vi "Two Lambda ZUP control panel.vi"() -> ()   [LabVIEW 2010]
uses:
  <vilib>/Instr/_visa.llb/VISA Configure Serial Port (Instr).vi
panel:
  in  "stop":bool
  out "Connected 2":bool
  out "Connected 1":bool
  in  "Run 2":bool
  in  "Run 1":bool
  out "read Lambda 2":string
  out "Code 2":string
  in  "Command 2":T1(ring)
  in  "Auxiliary Paramerter 2":dbl min=0.0 max=20.0 step=0.1
  out "read Lambda 1":string
  out "Code 1":string
  in  "Command 1":T1(ring)
  in  "Auxiliary Paramerter 1":dbl min=0.0 max=20.0 step=0.1
  in  "VISA resource name":refnum<visa-resource-name>
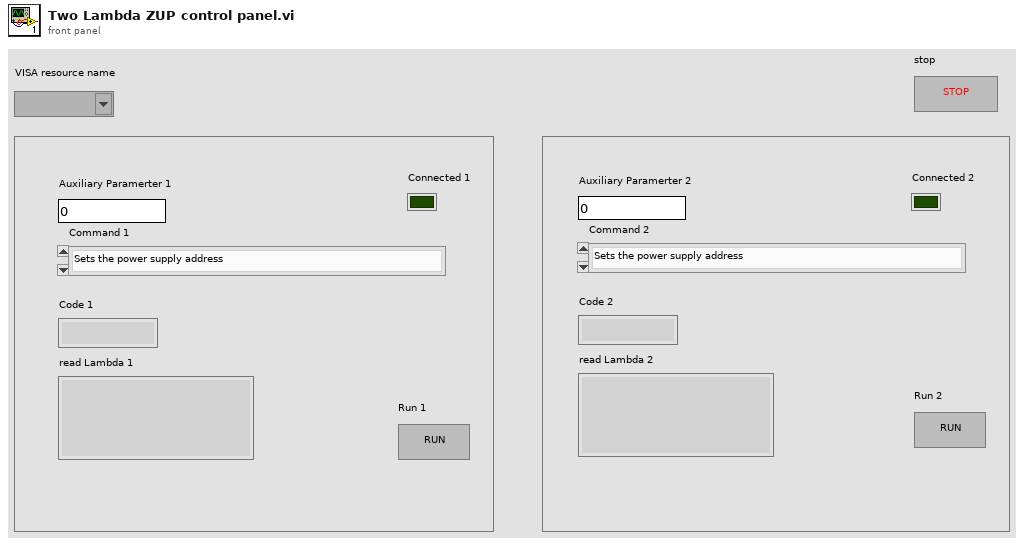
[diagram p1: front panel]
types:
  T1 = enum16{"Sets the power supply address", "Clears the communication buffer and the following registers", "Sets the power supply to local or remote mode", "Returns the remote/local setting", "Returns the power supply model identification", "Returns the software version", "Sets the output voltage value", "Returns the string SV (Set Voltage)", "Returns the string AV (Actual Voltage)", "Sets the output current in Ampers", "Returns the string SA (Set Amper)", "Returns the string AA (Actual Amper)", "Sets the output to On or Off", "Returns followed by the output On/Off status", "Sets the Foldback protection to On or Off", "Returns FD followed by the Foldback protection status", "Sets the over-voltage protection level in volts", "Returns the string OP  over-voltage protection value", "Sets the under-voltage protection limits in volts", "Returns the string UP under-voltage protection value", "Sets the auto-restart mode to On or Off", "Returns the string AS auto-restart mode status"}
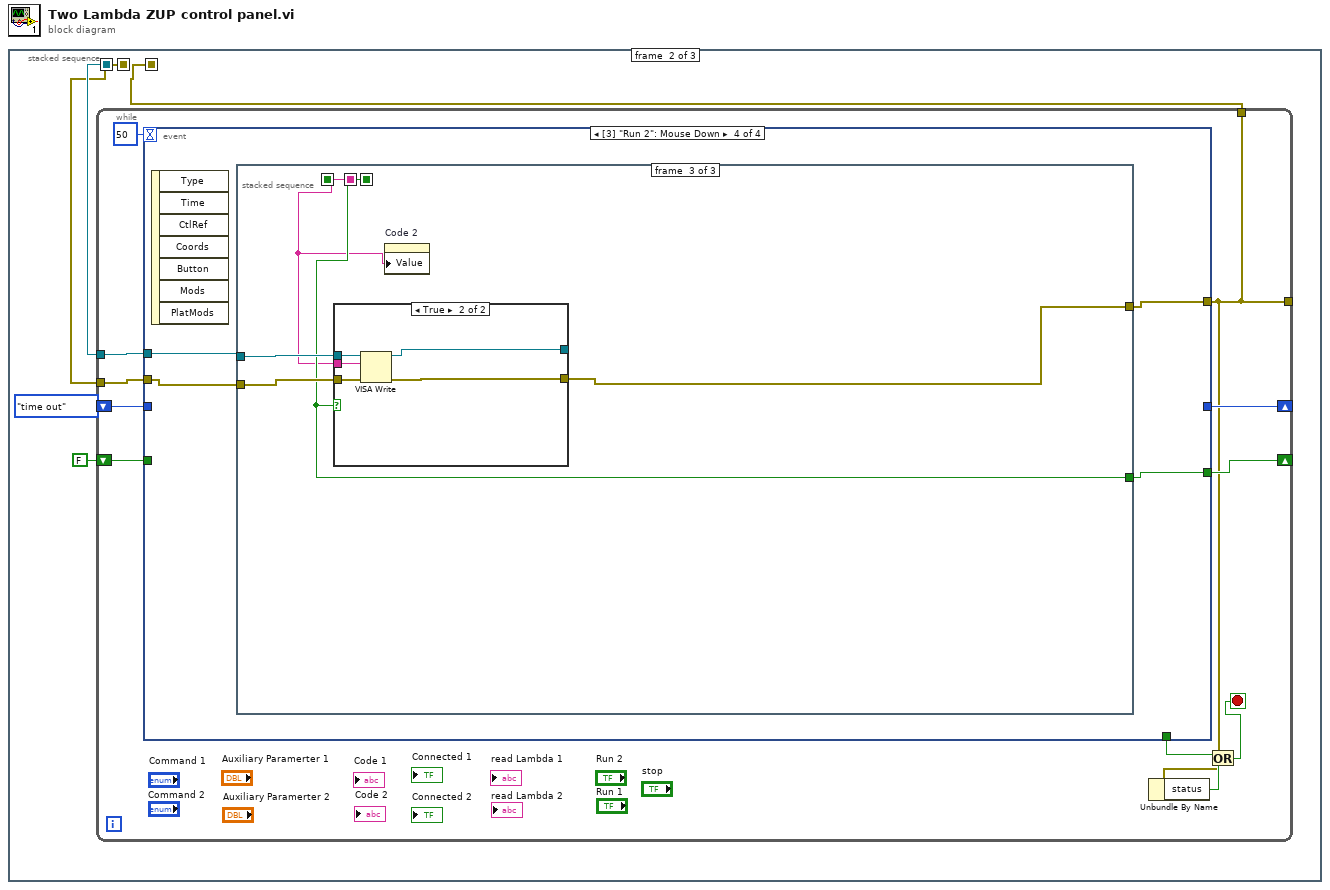
[diagram p0: block diagram]
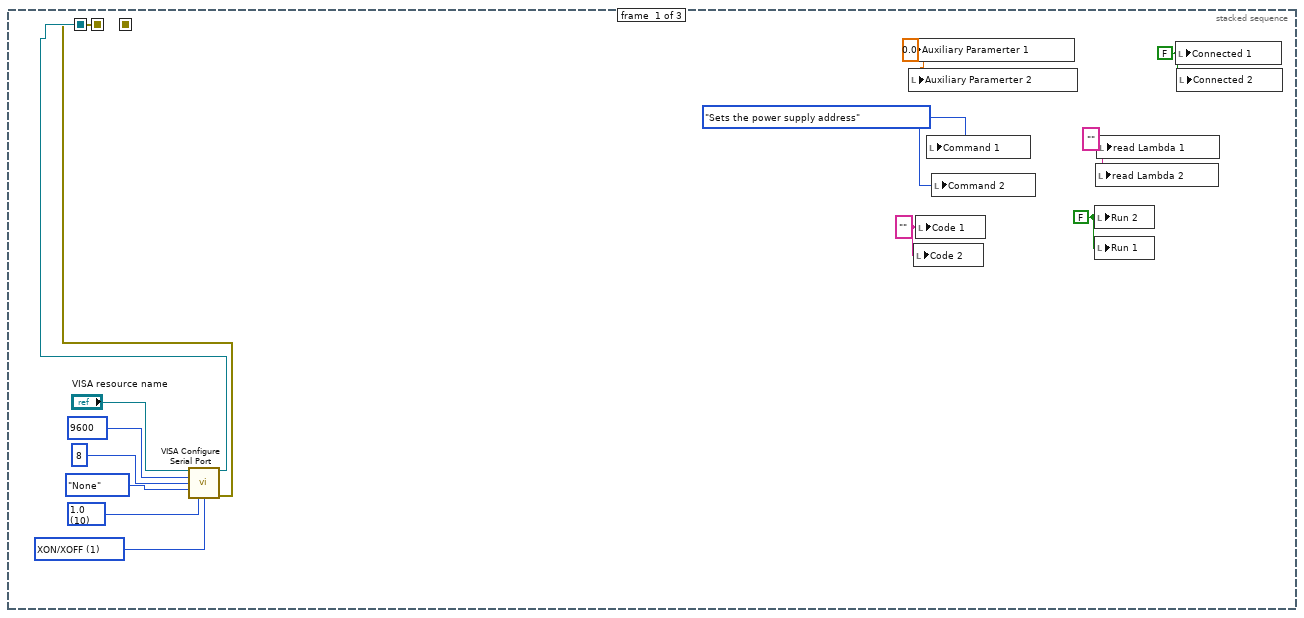
[diagram p2: hidden frame]
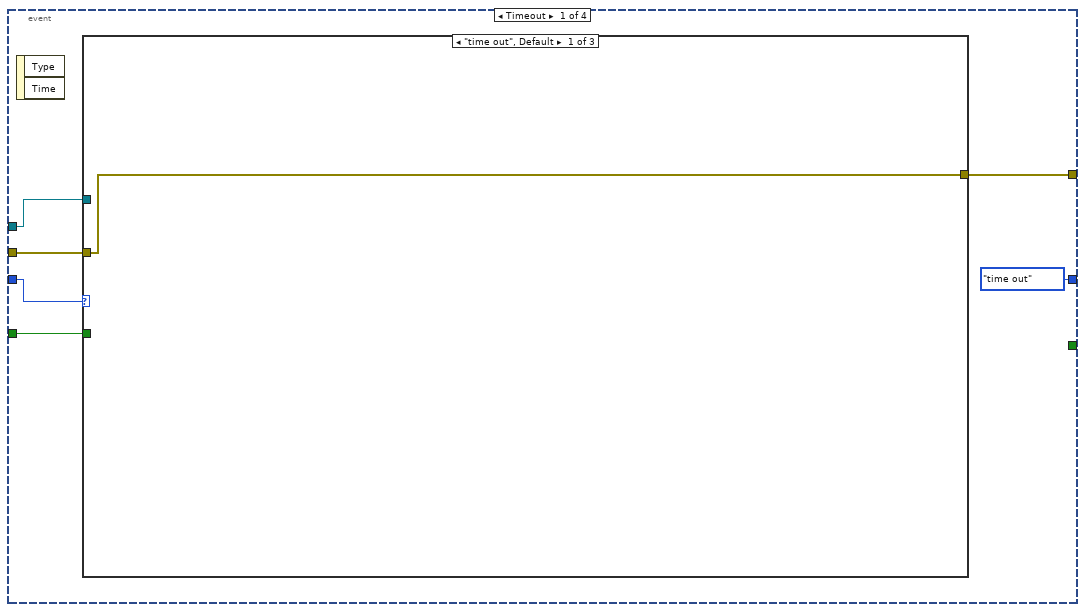
[diagram p3: hidden frame]
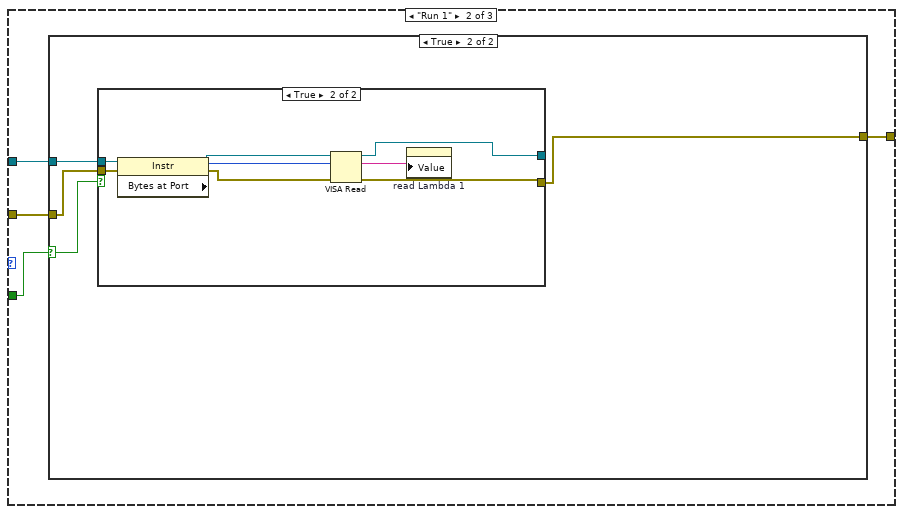
[diagram p4: hidden frame]
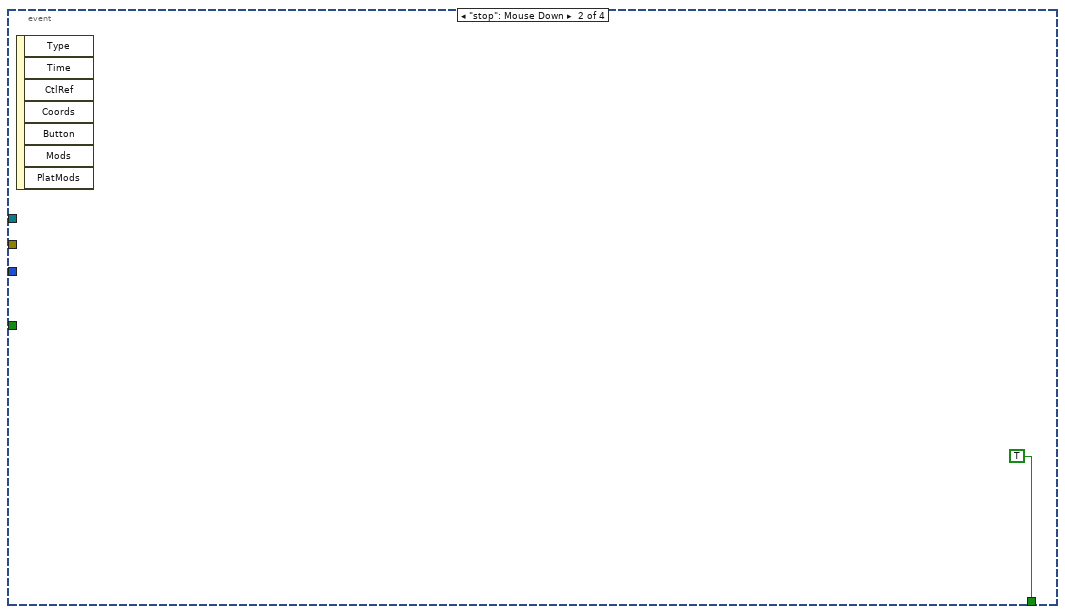
[diagram p8: hidden frame]
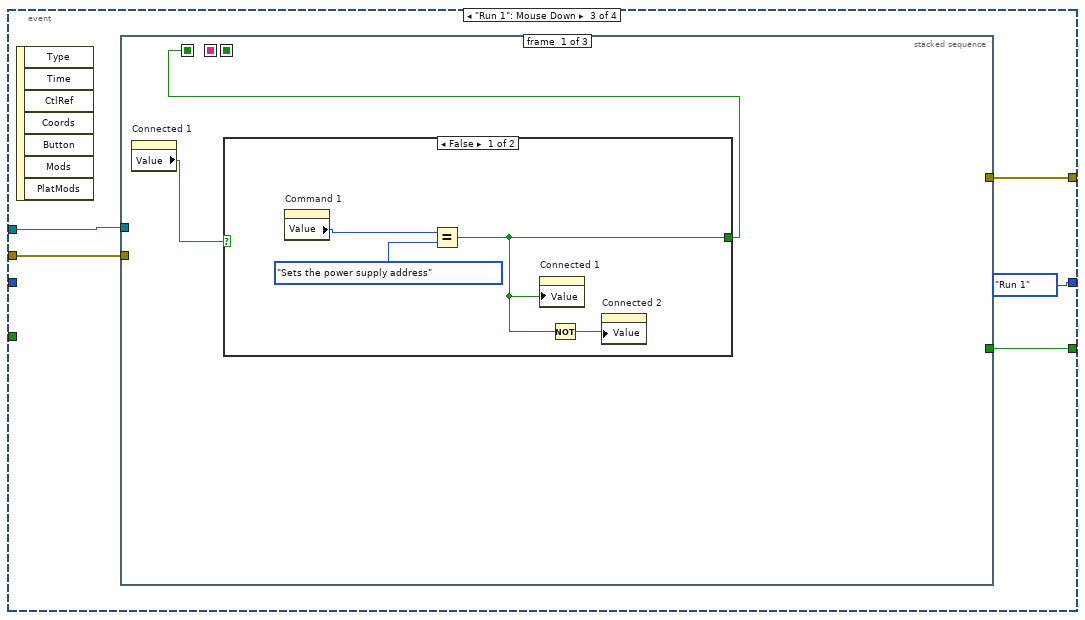
[diagram p9: hidden frame]
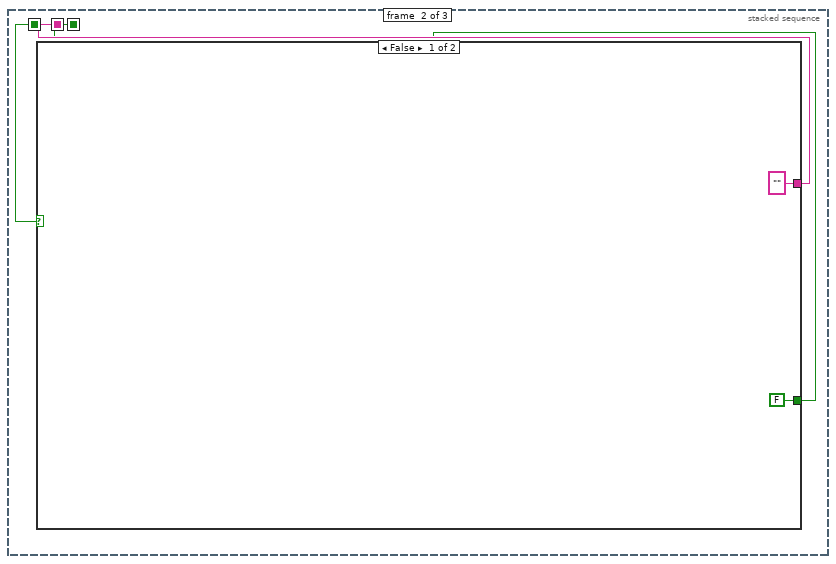
[diagram p11: hidden frame]
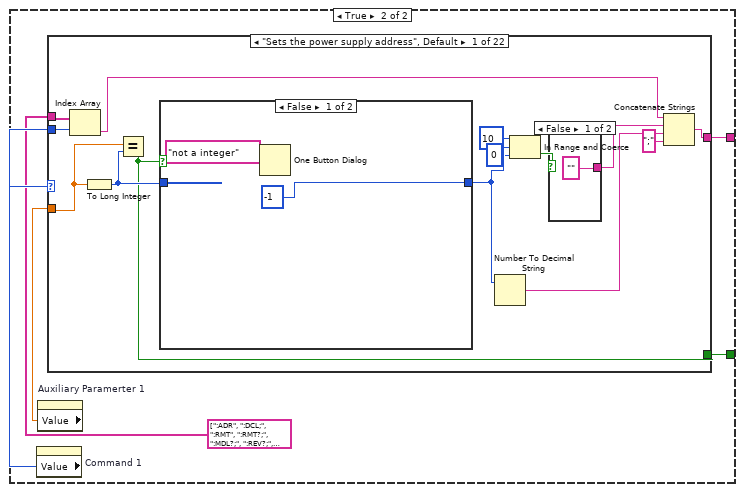
[diagram p12: hidden frame]
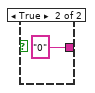
[diagram p13: hidden frame]
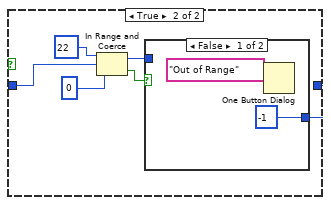
[diagram p14: hidden frame]
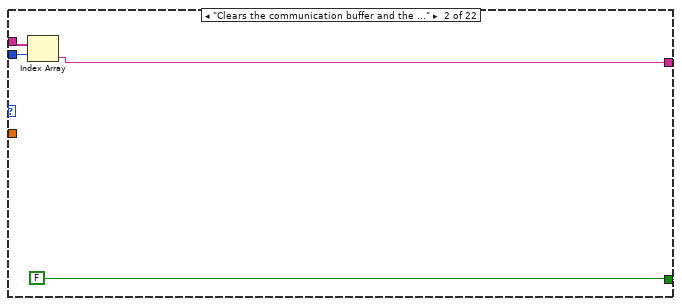
[diagram p16: hidden frame]
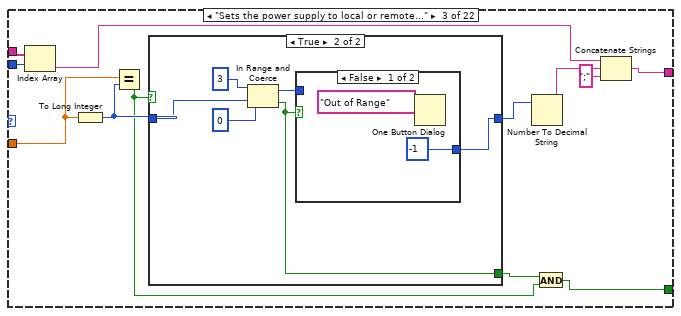
[diagram p17: hidden frame]
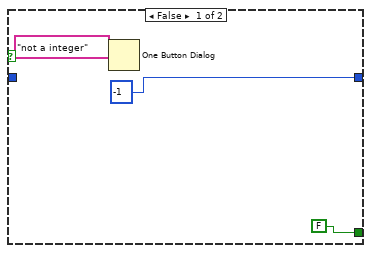
[diagram p18: hidden frame]
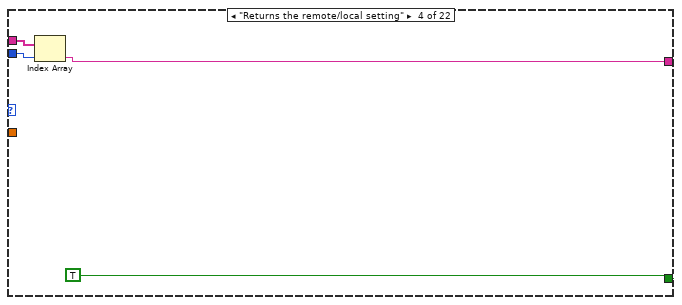
[diagram p20: hidden frame]
diagram:
  n1 = stacked-sequence {
    seq-local: [w2 _ _] -> [_ w19 w604]
    seq-local: [w1 _ _] -> [_ w18 _]
    seq-local: [_ w17 _] -> [_ _ w603]
    frame #0 {
      w4 = u16 1 items=["None", "XON/XOFF", "RTS/CTS", "XON/XOFF & RTS/CTS", "DTR/DSR", "XON/XOFF & DTR/DSR"] ("flow control (0:none)")
      w5 = u16 10 items=["1.0"=10, "1.5"=15, "2.0"=20] ("stop bits (10: 1 bit)")
      w9 = FALSE ("Run 2")
      w10 = "" ("read Lambda 1")
      w11 = "" ("Code 1")
      w12 = FALSE ("Connecting 1")
      w13 = T1."Sets the power supply address" ("Command")
      w14 = 0.0 ("Auxiliary Paramerter")
      n2 = call-poly "VISA Configure Serial Port"("VISA resource name"="VISA resource name", "baud rate (9600)"=u32 9600, "data bits (8)"=u16 8, "parity (0:none)"=enum16{"None", "Odd", "Even", "Mark", "Space"}."None", "stop bits (10: 1 bit)"=w5, "flow control (0:none)"=w4) -> ("VISA resource name out"=w2:refnum<visa-resource-name>, "error out"=w1:errorcluster)  [unwired: 8 in]
      n3 = local write "Auxiliary Paramerter 1"(w14) -> ()
      n4 = local write "Auxiliary Paramerter 2"(w14) -> ()
      n5 = local write "Code 2"(w11) -> ()
      n6 = local write "Code 1"(w11) -> ()
      n7 = local write "Command 1"(w13) -> ()
      n8 = local write "Command 2"(w13) -> ()
      n9 = local write "Run 2"(w9) -> ()
      n10 = local write "Run 1"(w9) -> ()
      n11 = local write "read Lambda 2"(w10) -> ()
      n12 = local write "read Lambda 1"(w10) -> ()
      n13 = local write "Connected 1"(w12) -> ()
      n14 = local write "Connected 2"(w12) -> ()
    }
    frame #1 {
      n15 = while {
        tunnel: w19 -> [w29]
        tunnel: w18 -> [w28]
        shift-right: [w27] -> _
        shift-left: enum16{"time out", "Run 1", "Run 2"}."time out" -> [w26]
        shift-right: [w22] -> _
        shift-left: FALSE -> [w21]
        tunnel: [w20] -> _
        tunnel: [w20] -> w17
        stop <- w23 stop-if-true
        n16 = event shown="[3] \"Run 2\": Mouse Down" {
          selector: _ -> [_ _ _ _]
          dyn-events: _ -> [_ _ _ _]
          timeout: 50 -> [_ _ _ _]
          tunnel: [_ TRUE _ _] -> w24
          tunnel: w29 -> [w34 _ w63 w334]
          tunnel: w28 -> [w33 _ w62 w333]
          tunnel: [enum16{"time out", "Run 1", "Run 2"}."time out" _ enum16{"time out", "Run 1", "Run 2"}."Run 1" _] -> w27
          tunnel: w26 -> [w36 _ _ _]
          tunnel: [w32 _ w60 w332] -> w20
          tunnel: [_ _ w59 w331] -> w22
          tunnel: w21 -> [w35 _ _ _]
          event Timeout {
            n17 = event-data() -> ()  [unwired: 1 in, 2 out]
            n18 = case shown="\"time out\", Default" w36 {
              tunnel: w35 -> [_ w41 _]
              tunnel: w34 -> [_ w40 _]
              tunnel: w33 -> [w37 w39 w57]
              tunnel: [w37 w38 w57] -> w32
              frame "time out", Default {
              }
              frame "Run 1" {
                n19 = case shown="True" w41 {
                  selector: w41 -> [_ w43]
                  tunnel: w40 -> [_ w46]
                  tunnel: w39 -> [w42 w45]
                  tunnel: [w42 w44] -> w38
                  frame False {
                  }
                  frame True {
                    n20 = case shown="True" w43 {
                      tunnel: w46 -> [w48 w56]
                      tunnel: w45 -> [w47 w55]
                      tunnel: [w48 w51] -> _
                      tunnel: [w47 w50] -> w44
                      frame False {
                      }
                      frame True {
                        n21 = property class="Instr"(reference=w56, error in=w55) -> (reference out=w54:refnum<visa-resource-name>, error out=w52:errorcluster, "Bytes at Port"=w53:u32)
                        n22 = VISA Read(VISA resource name=w54, byte count=w53, error in (no error)=w52) -> (VISA resource name out=w51:refnum<visa-resource-name>, read buffer=w49:string, error out=w50:errorcluster)  [unwired: 1 out]
                        n23 = property on="read Lambda 1" class="Str"("Value"=w49) -> ()  [unwired: 2 in, 2 out]
                      }
                    }
                  }
                }
              }
              frame "Run 2" {
              }
            }
          }
          event "stop": Mouse Down {
            n24 = event-data() -> ()  [unwired: 1 in, 7 out]
          }
          event "Run 1": Mouse Down {
            n25 = event-data() -> ()  [unwired: 1 in, 7 out]
            n26 = stacked-sequence {
              seq-local: [w64 _ _] -> [_ w73 _]
              seq-local: [_ w72 _] -> [_ _ w319]
              seq-local: [_ w71 _] -> [_ _ w320]
              tunnel: w63 -> [_ _ w323]
              tunnel: w62 -> [_ _ w322]
              tunnel: [_ _ w321] -> w60
              tunnel: [_ _ w320] -> w59
              frame #0 {
                n27 = property on="Connected 1" class="Bool (strict)"() -> ("Value"=w65:bool)  [unwired: 2 in, 2 out]
                n28 = case shown="False" w65 {
                  selector: w65 -> [_ w70]
                  tunnel: [w66 w70] -> w64
                  frame False {
                    n29 = property on="Command 1" class="Enum (strict)"() -> ("Value"=w68:T1)  [unwired: 2 in, 2 out]
                    n30 = Equal?(x=w68, y=T1."Sets the power supply address" ("Command 1")) -> (x = y?=w66:bool)
                    n31 = property on="Connected 1" class="Bool (strict)"("Value"=w66) -> ()  [unwired: 2 in, 2 out]
                    n32 = Not(x=w66) -> (.not. x?=w67:bool)
                    n33 = property on="Connected 2" class="Bool (strict)"("Value"=w67) -> ()  [unwired: 2 in, 2 out]
                  }
                  frame True {
                  }
                }
              }
              frame #1 {
                n34 = case shown="False" w73 {
                  tunnel: ["" w77] -> w72
                  tunnel: [FALSE w76] -> w71
                  frame False {
                  }
                  frame True {
                    n35 = property on="Command 1" class="Enum (strict)"() -> ("Value"=w79:T1)  [unwired: 2 in, 2 out]
                    n36 = property on="Auxiliary Paramerter 1" class="DigNum (strict)"() -> ("Value"=w80:dbl)  [unwired: 2 in, 2 out]
                    n37 = case shown="\"Sets the power supply address\", Default" w79 {
                      tunnel: w79 -> [w89 w111 w123 w139 w143 w147 w159 w165 w169 w177 w192 w196 w203 w224 w230 w252 w260 w271 w278 w289 w295 w318]
                      tunnel: string[] [":ADR", ":DCL;", ":RMT", ":RMT?;", ":MDL?;", ":REV?;", ":VOL", ":VOL!;", ":VOL?;", ":CUR", ":CUR!;", ":CUR?;", ":OUT", ":OUT?;", ":FLD", ":FLD?;", ":OVP", ":OVP?;", ":UVP", ":UVP?;", ":AST", ":AST?;"] -> [w90 w110 w122 w138 w142 w146 w160 w166 w170 w178 w191 w195 w202 w223 w231 w251 w259 w270 w279 w290 w296 w317]
                      tunnel: [w88 w109 w116 w137 w141 w145 w158 w164 w168 w174 w190 w194 w200 w222 w228 w250 w258 w269 w277 w288 w294 w316] -> w77
                      tunnel: w80 -> [w91 _ w115 _ _ _ w152 _ _ w182 _ _ w204 _ w229 _ w257 _ w276 _ w297 _]
                      tunnel: [w81 FALSE w112 TRUE TRUE TRUE TRUE TRUE TRUE w171 TRUE TRUE w197 TRUE w225 TRUE TRUE TRUE TRUE TRUE w291 TRUE] -> w76
                      frame "Sets the power supply address", Default {
                        n38 = Index Array(array=w90, index=w89) -> (element=w82:string)
                        n39 = To Long Integer(number=w91) -> (32bit integer=w94:i32)
                        n40 = Equal?(x=w91, y=w94) -> (x = y?=w81:bool)
                        n41 = case shown="False" w81 {
                          tunnel: w94 -> [_ w101]
                          tunnel: [-1 w100] -> w87
                          frame False {
                            n42 = One Button Dialog(message="not a integer") -> ()  [unwired: 1 in, 1 out]
                          }
                          frame True {
                            n43 = In Range and Coerce(upper limit=22, x=w101, lower limit=0) -> (coerced(x)=w99:i32, In Range?=w104:bool)
                            n44 = case shown="False" w104 {
                              tunnel: [-1 w107] -> w100
                              tunnel: w99 -> [_ w107]
                              frame False {
                                n45 = One Button Dialog(message="Out of Range") -> ()  [unwired: 1 in, 1 out]
                              }
                              frame True {
                              }
                            }
                          }
                        }
                        n46 = Number To Decimal String(number=w87) -> (decimal integer string=w93:string)  [unwired: 1 in]
                        n47 = In Range and Coerce(upper limit=10, x=w87, lower limit=0) -> (In Range?=w84:bool)  [unwired: 1 out]
                        n48 = case shown="False" w84 {
                          tunnel: ["" "0"] -> w83
                          frame False {
                          }
                          frame True {
                          }
                        }
                        n49 = Concatenate Strings(w82, w83, w93, ";" ("string")) -> (w88:string)
                      }
                      frame "Clears the communication buffer and the following registers" {
                        n50 = Index Array(array=w110, index=w111) -> (element=w109:string)
                      }
                      frame "Sets the power supply to local or remote mode" {
                        n51 = Index Array(array=w122, index=w123) -> (element=w119:string)
                        n52 = To Long Integer(number=w115) -> (32bit integer=w121:i32)
                        n53 = Equal?(x=w115, y=w121) -> (x = y?=w114:bool)
                        n54 = case shown="True" w114 {
                          tunnel: w121 -> [_ w130]
                          tunnel: [-1 w129] -> w120
                          tunnel: [FALSE w127] -> w113
                          frame False {
                            n55 = One Button Dialog(message="not a integer") -> ()  [unwired: 1 in, 1 out]
                          }
                          frame True {
                            n56 = In Range and Coerce(upper limit=3, x=w130, lower limit=0) -> (coerced(x)=w128:i32, In Range?=w127:bool)
                            n57 = case shown="False" w127 {
                              tunnel: [-1 w135] -> w129
                              tunnel: w128 -> [_ w135]
                              frame False {
                                n58 = One Button Dialog(message="Out of Range") -> ()  [unwired: 1 in, 1 out]
                              }
                              frame True {
                              }
                            }
                          }
                        }
                        n59 = Number To Decimal String(number=w120) -> (decimal integer string=w118:string)  [unwired: 1 in]
                        n60 = And(x=w113, y=w114) -> (x .and. y?=w112:bool)
                        n61 = Concatenate Strings(w119, w118, ";" ("string")) -> (w116:string)
                      }
                      frame "Returns the remote/local setting" {
                        n62 = Index Array(array=w138, index=w139) -> (element=w137:string)
                      }
                      frame "Returns the power supply model identification" {
                        n63 = Index Array(array=w142, index=w143) -> (element=w141:string)
                      }
                      frame "Returns the software version" {
                        n64 = Index Array(array=w146, index=w147) -> (element=w145:string)
                      }
                      frame "Sets the output voltage value" {
                        n65 = Index Array(array=w160, index=w159) -> (element=w153:string)
                        n66 = Number To Fractional String(number=w152, width (-)=i16 4, precision (6)=i16 3) -> (F-format string=w156:string)  [unwired: 1 in]
                        n67 = Greater Or Equal?(x=w152, y=10.0) -> (x >= y?=w150:bool)
                        n68 = case shown="False" w150 {
                          tunnel: ["0" ("string") ""] -> w149
                          frame False {
                          }
                          frame True {
                          }
                        }
                        n69 = Concatenate Strings(w153, w149, w156, ";" ("string")) -> (w158:string)
                      }
                      frame "Returns the string SV (Set Voltage)" {
                        n70 = Index Array(array=w166, index=w165) -> (element=w164:string)
                      }
                      frame "Returns the string AV (Actual Voltage)" {
                        n71 = Index Array(array=w170, index=w169) -> (element=w168:string)
                      }
                      frame "Sets the output current in Ampers" {
                        n72 = Index Array(array=w178, index=w177) -> (element=w173:string)
                        n73 = In Range and Coerce(upper limit=10.0, x=w182, lower limit=0.0) -> (coerced(x)=w179:dbl, In Range?=w171:bool)
                        n74 = case shown="False" w171 {
                          tunnel: w179 -> [_ w188]
                          tunnel: ["-1" w185] -> w176
                          frame False {
                            n75 = One Button Dialog(message="Out of Range") -> ()  [unwired: 1 in, 1 out]
                          }
                          frame True {
                            n76 = Number To Fractional String(number=w188, width (-)=i16 4, precision (6)=i16 3) -> (F-format string=w185:string)  [unwired: 1 in]
                          }
                        }
                        n77 = Concatenate Strings(w173, "0" ("string"), w176, ";" ("string")) -> (w174:string)
                      }
                      frame "Returns the string SA (Set Amper)" {
                        n78 = Index Array(array=w191, index=w192) -> (element=w190:string)
                      }
                      frame "Returns the string AA (Actual Amper)" {
                        n79 = Index Array(array=w195, index=w196) -> (element=w194:string)
                      }
                      frame "Sets the output to On or Off" {
                        n80 = Index Array(array=w202, index=w203) -> (element=w201:string)
                        n81 = To Long Integer(number=w204) -> (32bit integer=w208:i32)
                        n82 = Equal?(x=w204, y=w208) -> (x = y?=w199:bool)
                        n83 = case shown="True" w199 {
                          tunnel: w208 -> [_ w215]
                          tunnel: [-1 w214] -> w207
                          tunnel: [FALSE w212] -> w198
                          frame False {
                            n84 = One Button Dialog(message="not a integer") -> ()  [unwired: 1 in, 1 out]
                          }
                          frame True {
                            n85 = In Range and Coerce(upper limit=2, x=w215, lower limit=-1) -> (coerced(x)=w213:i32, In Range?=w212:bool)
                            n86 = case shown="False" w212 {
                              tunnel: [-1 w220] -> w214
                              tunnel: w213 -> [_ w220]
                              frame False {
                                n87 = One Button Dialog(message="Out of Range") -> ()  [unwired: 1 in, 1 out]
                              }
                              frame True {
                              }
                            }
                          }
                        }
                        n88 = And(x=w198, y=w199) -> (x .and. y?=w197:bool)
                        n89 = Number To Decimal String(number=w207) -> (decimal integer string=w206:string)  [unwired: 1 in]
                        n90 = Concatenate Strings(w201, w206, ";" ("string")) -> (w200:string)
                      }
                      frame "Returns followed by the output On/Off status" {
                        n91 = Index Array(array=w223, index=w224) -> (element=w222:string)
                      }
                      frame "Sets the Foldback protection to On or Off" {
                        n92 = Index Array(array=w231, index=w230) -> (element=w234:string)
                        n93 = To Long Integer(number=w229) -> (32bit integer=w236:i32)
                        n94 = Equal?(x=w229, y=w236) -> (x = y?=w227:bool)
                        n95 = case shown="True" w227 {
                          tunnel: w236 -> [_ w243]
                          tunnel: [-1 w242] -> w235
                          tunnel: [FALSE w240] -> w226
                          frame False {
                            n96 = One Button Dialog(message="not a integer") -> ()  [unwired: 1 in, 1 out]
                          }
                          frame True {
                            n97 = In Range and Coerce(upper limit=2, x=w243, lower limit=0) -> (coerced(x)=w241:i32, In Range?=w240:bool)
                            n98 = case shown="False" w240 {
                              tunnel: [-1 w248] -> w242
                              tunnel: w241 -> [_ w248]
                              frame False {
                                n99 = One Button Dialog(message="Out of Range") -> ()  [unwired: 1 in, 1 out]
                              }
                              frame True {
                              }
                            }
                          }
                        }
                        n100 = And(x=w226, y=w227) -> (x .and. y?=w225:bool)
                        n101 = Number To Decimal String(number=w235) -> (decimal integer string=w233:string)  [unwired: 1 in]
                        n102 = Concatenate Strings(w234, w233, ";" ("string")) -> (w228:string)
                      }
                      frame "Returns FD followed by the Foldback protection status" {
                        n103 = Index Array(array=w251, index=w252) -> (element=w250:string)
                      }
                      frame "Sets the over-voltage protection level in volts" {
                        n104 = Index Array(array=w259, index=w260) -> (element=w261:string)
                        n105 = Number To Fractional String(number=w257, width (-)=i16 4, precision (6)=i16 3) -> (F-format string=w264:string)  [unwired: 1 in]
                        n106 = Greater Or Equal?(x=w257, y=10.0) -> (x >= y?=w255:bool)
                        n107 = case shown="True" w255 {
                          tunnel: ["0" ("string") ""] -> w254
                          frame False {
                          }
                          frame True {
                          }
                        }
                        n108 = Concatenate Strings(w261, w254, w264, ";" ("string")) -> (w258:string)
                      }
                      frame "Returns the string OP  over-voltage protection value" {
                        n109 = Index Array(array=w270, index=w271) -> (element=w269:string)
                      }
                      frame "Sets the under-voltage protection limits in volts" {
                        n110 = Index Array(array=w279, index=w278) -> (element=w280:string)
                        n111 = Number To Fractional String(number=w276, width (-)=i16 4, precision (6)=i16 3) -> (F-format string=w283:string)  [unwired: 1 in]
                        n112 = Greater Or Equal?(x=w276, y=10.0) -> (x >= y?=w274:bool)
                        n113 = case shown="True" w274 {
                          tunnel: ["0" ("string") ""] -> w273
                          frame False {
                          }
                          frame True {
                          }
                        }
                        n114 = Concatenate Strings(w280, w273, w283, ";" ("string")) -> (w277:string)
                      }
                      frame "Returns the string UP under-voltage protection value" {
                        n115 = Index Array(array=w290, index=w289) -> (element=w288:string)
                      }
                      frame "Sets the auto-restart mode to On or Off" {
                        n116 = Index Array(array=w296, index=w295) -> (element=w300:string)
                        n117 = To Long Integer(number=w297) -> (32bit integer=w302:i32)
                        n118 = Equal?(x=w297, y=w302) -> (x = y?=w293:bool)
                        n119 = case shown="False" w293 {
                          tunnel: w302 -> [_ w309]
                          tunnel: [-1 w308] -> w301
                          tunnel: [FALSE w306] -> w292
                          frame False {
                            n120 = One Button Dialog(message="not a integer") -> ()  [unwired: 1 in, 1 out]
                          }
                          frame True {
                            n121 = In Range and Coerce(upper limit=2, x=w309, lower limit=0) -> (coerced(x)=w307:i32, In Range?=w306:bool)
                            n122 = case shown="False" w306 {
                              tunnel: [-1 w314] -> w308
                              tunnel: w307 -> [_ w314]
                              frame False {
                                n123 = One Button Dialog(message="Out of Range") -> ()  [unwired: 1 in, 1 out]
                              }
                              frame True {
                              }
                            }
                          }
                        }
                        n124 = And(x=w292, y=w293) -> (x .and. y?=w291:bool)
                        n125 = Number To Decimal String(number=w301) -> (decimal integer string=w299:string)  [unwired: 1 in]
                        n126 = Concatenate Strings(w300, w299, ";" ("string")) -> (w294:string)
                      }
                      frame "Returns the string AS auto-restart mode status" {
                        n127 = Index Array(array=w317, index=w318) -> (element=w316:string)
                      }
                    }
                  }
                }
              }
              frame #2 {
                n128 = case shown="True" w320 {
                  tunnel: w323 -> [w325 w330]
                  tunnel: w322 -> [w324 w329]
                  tunnel: w319 -> [_ w328]
                  tunnel: [w325 w327] -> _
                  tunnel: [w324 w326] -> w321
                  frame False {
                  }
                  frame True {
                    n129 = VISA Write(VISA resource name=w330, write buffer=w328, error in (no error)=w329) -> (VISA resource name out=w327:refnum<visa-resource-name>, error out=w326:errorcluster)  [unwired: 1 out]
                  }
                }
                n130 = property on="Code 1" class="Str"("Value"=w319) -> ()  [unwired: 2 in, 2 out]
              }
            }
          }
          event "Run 2": Mouse Down {
            n131 = event-data() -> ()  [unwired: 1 in, 7 out]
            n132 = stacked-sequence {
              seq-local: [w335 _ _] -> [_ w344 _]
              seq-local: [_ w343 _] -> [_ _ w590]
              seq-local: [_ w342 _] -> [_ _ w591]
              tunnel: w334 -> [_ _ w594]
              tunnel: w333 -> [_ _ w593]
              tunnel: [_ _ w592] -> w332
              tunnel: [_ _ w591] -> w331
              frame #0 {
                n133 = property on="Connected 2" class="Bool (strict)"() -> ("Value"=w336:bool)  [unwired: 2 in, 2 out]
                n134 = case shown="True" w336 {
                  selector: w336 -> [_ w341]
                  tunnel: [w337 w341] -> w335
                  frame False {
                    n135 = property on="Command 2" class="Enum (strict)"() -> ("Value"=w339:T1)  [unwired: 2 in, 2 out]
                    n136 = Equal?(x=w339, y=T1."Sets the power supply address" ("Command 1")) -> (x = y?=w337:bool)
                    n137 = Not(x=w337) -> (.not. x?=w338:bool)
                    n138 = property on="Connected 2" class="Bool (strict)"("Value"=w337) -> ()  [unwired: 2 in, 2 out]
                    n139 = property on="Connected 1" class="Bool (strict)"("Value"=w338) -> ()  [unwired: 2 in, 2 out]
                  }
                  frame True {
                  }
                }
              }
              frame #1 {
                n140 = case shown="True" w344 {
                  tunnel: ["" w348] -> w343
                  tunnel: [FALSE w347] -> w342
                  frame False {
                  }
                  frame True {
                    n141 = property on="Command 2" class="Enum (strict)"() -> ("Value"=w350:T1)  [unwired: 2 in, 2 out]
                    n142 = property on="Auxiliary Paramerter 2" class="DigNum (strict)"() -> ("Value"=w351:dbl)  [unwired: 2 in, 2 out]
                    n143 = case shown="\"Sets the power supply address\", Default" w350 {
                      tunnel: w350 -> [w360 w382 w394 w410 w414 w418 w430 w436 w440 w448 w463 w467 w474 w495 w501 w523 w531 w542 w549 w560 w566 w589]
                      tunnel: string[] [":ADR", ":DCL;", ":RMT", ":RMT?;", ":MDL?;", ":REV?;", ":VOL", ":VOL!;", ":VOL?;", ":CUR", ":CUR!;", ":CUR?;", ":OUT", ":OUT?;", ":FLD", ":FLD?;", ":OVP", ":OVP?;", ":UVP", ":UVP?;", ":AST", ":AST?;"] -> [w361 w381 w393 w409 w413 w417 w431 w437 w441 w449 w462 w466 w473 w494 w502 w522 w530 w541 w550 w561 w567 w588]
                      tunnel: [w359 w380 w387 w408 w412 w416 w429 w435 w439 w445 w461 w465 w471 w493 w499 w521 w529 w540 w548 w559 w565 w587] -> w348
                      tunnel: w351 -> [w362 _ w386 _ _ _ w423 _ _ w453 _ _ w475 _ w500 _ w528 _ w547 _ w568 _]
                      tunnel: [w352 FALSE w383 TRUE TRUE TRUE TRUE TRUE TRUE w442 TRUE TRUE w468 TRUE w496 TRUE TRUE TRUE TRUE TRUE w562 TRUE] -> w347
                      frame "Sets the power supply address", Default {
                        n144 = Index Array(array=w361, index=w360) -> (element=w353:string)
                        n145 = To Long Integer(number=w362) -> (32bit integer=w365:i32)
                        n146 = Equal?(x=w362, y=w365) -> (x = y?=w352:bool)
                        n147 = case shown="False" w352 {
                          tunnel: w365 -> [_ w372]
                          tunnel: [-1 w371] -> w358
                          frame False {
                            n148 = One Button Dialog(message="not a integer") -> ()  [unwired: 1 in, 1 out]
                          }
                          frame True {
                            n149 = In Range and Coerce(upper limit=22, x=w372, lower limit=0) -> (coerced(x)=w370:i32, In Range?=w375:bool)
                            n150 = case shown="False" w375 {
                              tunnel: [-1 w378] -> w371
                              tunnel: w370 -> [_ w378]
                              frame False {
                                n151 = One Button Dialog(message="Out of Range") -> ()  [unwired: 1 in, 1 out]
                              }
                              frame True {
                              }
                            }
                          }
                        }
                        n152 = Number To Decimal String(number=w358) -> (decimal integer string=w364:string)  [unwired: 1 in]
                        n153 = In Range and Coerce(upper limit=10, x=w358, lower limit=0) -> (In Range?=w355:bool)  [unwired: 1 out]
                        n154 = case shown="False" w355 {
                          tunnel: ["" "0"] -> w354
                          frame False {
                          }
                          frame True {
                          }
                        }
                        n155 = Concatenate Strings(w353, w354, w364, ";" ("string")) -> (w359:string)
                      }
                      frame "Clears the communication buffer and the following registers" {
                        n156 = Index Array(array=w381, index=w382) -> (element=w380:string)
                      }
                      frame "Sets the power supply to local or remote mode" {
                        n157 = Index Array(array=w393, index=w394) -> (element=w390:string)
                        n158 = To Long Integer(number=w386) -> (32bit integer=w392:i32)
                        n159 = Equal?(x=w386, y=w392) -> (x = y?=w385:bool)
                        n160 = case shown="True" w385 {
                          tunnel: w392 -> [_ w401]
                          tunnel: [-1 w400] -> w391
                          tunnel: [FALSE w398] -> w384
                          frame False {
                            n161 = One Button Dialog(message="not a integer") -> ()  [unwired: 1 in, 1 out]
                          }
                          frame True {
                            n162 = In Range and Coerce(upper limit=3, x=w401, lower limit=0) -> (coerced(x)=w399:i32, In Range?=w398:bool)
                            n163 = case shown="False" w398 {
                              tunnel: [-1 w406] -> w400
                              tunnel: w399 -> [_ w406]
                              frame False {
                                n164 = One Button Dialog(message="Out of Range") -> ()  [unwired: 1 in, 1 out]
                              }
                              frame True {
                              }
                            }
                          }
                        }
                        n165 = Number To Decimal String(number=w391) -> (decimal integer string=w389:string)  [unwired: 1 in]
                        n166 = And(x=w384, y=w385) -> (x .and. y?=w383:bool)
                        n167 = Concatenate Strings(w390, w389, ";" ("string")) -> (w387:string)
                      }
                      frame "Returns the remote/local setting" {
                        n168 = Index Array(array=w409, index=w410) -> (element=w408:string)
                      }
                      frame "Returns the power supply model identification" {
                        n169 = Index Array(array=w413, index=w414) -> (element=w412:string)
                      }
                      frame "Returns the software version" {
                        n170 = Index Array(array=w417, index=w418) -> (element=w416:string)
                      }
                      frame "Sets the output voltage value" {
                        n171 = Index Array(array=w431, index=w430) -> (element=w424:string)
                        n172 = Number To Fractional String(number=w423, width (-)=i16 4, precision (6)=i16 3) -> (F-format string=w427:string)  [unwired: 1 in]
                        n173 = Greater Or Equal?(x=w423, y=10.0) -> (x >= y?=w421:bool)
                        n174 = case shown="False" w421 {
                          tunnel: ["0" ("string") ""] -> w420
                          frame False {
                          }
                          frame True {
                          }
                        }
                        n175 = Concatenate Strings(w424, w420, w427, ";" ("string")) -> (w429:string)
                      }
                      frame "Returns the string SV (Set Voltage)" {
                        n176 = Index Array(array=w437, index=w436) -> (element=w435:string)
                      }
                      frame "Returns the string AV (Actual Voltage)" {
                        n177 = Index Array(array=w441, index=w440) -> (element=w439:string)
                      }
                      frame "Sets the output current in Ampers" {
                        n178 = Index Array(array=w449, index=w448) -> (element=w444:string)
                        n179 = In Range and Coerce(upper limit=10.0, x=w453, lower limit=0.0) -> (coerced(x)=w450:dbl, In Range?=w442:bool)
                        n180 = case shown="False" w442 {
                          tunnel: w450 -> [_ w459]
                          tunnel: ["-1" w456] -> w447
                          frame False {
                            n181 = One Button Dialog(message="Out of Range") -> ()  [unwired: 1 in, 1 out]
                          }
                          frame True {
                            n182 = Number To Fractional String(number=w459, width (-)=i16 4, precision (6)=i16 3) -> (F-format string=w456:string)  [unwired: 1 in]
                          }
                        }
                        n183 = Concatenate Strings(w444, "0" ("string"), w447, ";" ("string")) -> (w445:string)
                      }
                      frame "Returns the string SA (Set Amper)" {
                        n184 = Index Array(array=w462, index=w463) -> (element=w461:string)
                      }
                      frame "Returns the string AA (Actual Amper)" {
                        n185 = Index Array(array=w466, index=w467) -> (element=w465:string)
                      }
                      frame "Sets the output to On or Off" {
                        n186 = Index Array(array=w473, index=w474) -> (element=w472:string)
                        n187 = To Long Integer(number=w475) -> (32bit integer=w479:i32)
                        n188 = Equal?(x=w475, y=w479) -> (x = y?=w470:bool)
                        n189 = case shown="True" w470 {
                          tunnel: w479 -> [_ w486]
                          tunnel: [-1 w485] -> w478
                          tunnel: [FALSE w483] -> w469
                          frame False {
                            n190 = One Button Dialog(message="not a integer") -> ()  [unwired: 1 in, 1 out]
                          }
                          frame True {
                            n191 = In Range and Coerce(upper limit=2, x=w486, lower limit=-1) -> (coerced(x)=w484:i32, In Range?=w483:bool)
                            n192 = case shown="False" w483 {
                              tunnel: [-1 w491] -> w485
                              tunnel: w484 -> [_ w491]
                              frame False {
                                n193 = One Button Dialog(message="Out of Range") -> ()  [unwired: 1 in, 1 out]
                              }
                              frame True {
                              }
                            }
                          }
                        }
                        n194 = And(x=w469, y=w470) -> (x .and. y?=w468:bool)
                        n195 = Number To Decimal String(number=w478) -> (decimal integer string=w477:string)  [unwired: 1 in]
                        n196 = Concatenate Strings(w472, w477, ";" ("string")) -> (w471:string)
                      }
                      frame "Returns followed by the output On/Off status" {
                        n197 = Index Array(array=w494, index=w495) -> (element=w493:string)
                      }
                      frame "Sets the Foldback protection to On or Off" {
                        n198 = Index Array(array=w502, index=w501) -> (element=w505:string)
                        n199 = To Long Integer(number=w500) -> (32bit integer=w507:i32)
                        n200 = Equal?(x=w500, y=w507) -> (x = y?=w498:bool)
                        n201 = case shown="True" w498 {
                          tunnel: w507 -> [_ w514]
                          tunnel: [-1 w513] -> w506
                          tunnel: [FALSE w511] -> w497
                          frame False {
                            n202 = One Button Dialog(message="not a integer") -> ()  [unwired: 1 in, 1 out]
                          }
                          frame True {
                            n203 = In Range and Coerce(upper limit=2, x=w514, lower limit=0) -> (coerced(x)=w512:i32, In Range?=w511:bool)
                            n204 = case shown="False" w511 {
                              tunnel: [-1 w519] -> w513
                              tunnel: w512 -> [_ w519]
                              frame False {
                                n205 = One Button Dialog(message="Out of Range") -> ()  [unwired: 1 in, 1 out]
                              }
                              frame True {
                              }
                            }
                          }
                        }
                        n206 = And(x=w497, y=w498) -> (x .and. y?=w496:bool)
                        n207 = Number To Decimal String(number=w506) -> (decimal integer string=w504:string)  [unwired: 1 in]
                        n208 = Concatenate Strings(w505, w504, ";" ("string")) -> (w499:string)
                      }
                      frame "Returns FD followed by the Foldback protection status" {
                        n209 = Index Array(array=w522, index=w523) -> (element=w521:string)
                      }
                      frame "Sets the over-voltage protection level in volts" {
                        n210 = Index Array(array=w530, index=w531) -> (element=w532:string)
                        n211 = Number To Fractional String(number=w528, width (-)=i16 4, precision (6)=i16 3) -> (F-format string=w535:string)  [unwired: 1 in]
                        n212 = Greater Or Equal?(x=w528, y=10.0) -> (x >= y?=w526:bool)
                        n213 = case shown="True" w526 {
                          tunnel: ["0" ("string") ""] -> w525
                          frame False {
                          }
                          frame True {
                          }
                        }
                        n214 = Concatenate Strings(w532, w525, w535, ";" ("string")) -> (w529:string)
                      }
                      frame "Returns the string OP  over-voltage protection value" {
                        n215 = Index Array(array=w541, index=w542) -> (element=w540:string)
                      }
                      frame "Sets the under-voltage protection limits in volts" {
                        n216 = Index Array(array=w550, index=w549) -> (element=w551:string)
                        n217 = Number To Fractional String(number=w547, width (-)=i16 4, precision (6)=i16 3) -> (F-format string=w554:string)  [unwired: 1 in]
                        n218 = Greater Or Equal?(x=w547, y=10.0) -> (x >= y?=w545:bool)
                        n219 = case shown="True" w545 {
                          tunnel: ["0" ("string") ""] -> w544
                          frame False {
                          }
                          frame True {
                          }
                        }
                        n220 = Concatenate Strings(w551, w544, w554, ";" ("string")) -> (w548:string)
                      }
                      frame "Returns the string UP under-voltage protection value" {
                        n221 = Index Array(array=w561, index=w560) -> (element=w559:string)
                      }
                      frame "Sets the auto-restart mode to On or Off" {
                        n222 = Index Array(array=w567, index=w566) -> (element=w571:string)
                        n223 = To Long Integer(number=w568) -> (32bit integer=w573:i32)
                        n224 = Equal?(x=w568, y=w573) -> (x = y?=w564:bool)
                        n225 = case shown="False" w564 {
                          tunnel: w573 -> [_ w580]
                          tunnel: [-1 w579] -> w572
                          tunnel: [FALSE w577] -> w563
                          frame False {
                            n226 = One Button Dialog(message="not a integer") -> ()  [unwired: 1 in, 1 out]
                          }
                          frame True {
                            n227 = In Range and Coerce(upper limit=2, x=w580, lower limit=0) -> (coerced(x)=w578:i32, In Range?=w577:bool)
                            n228 = case shown="False" w577 {
                              tunnel: [-1 w585] -> w579
                              tunnel: w578 -> [_ w585]
                              frame False {
                                n229 = One Button Dialog(message="Out of Range") -> ()  [unwired: 1 in, 1 out]
                              }
                              frame True {
                              }
                            }
                          }
                        }
                        n230 = And(x=w563, y=w564) -> (x .and. y?=w562:bool)
                        n231 = Number To Decimal String(number=w572) -> (decimal integer string=w570:string)  [unwired: 1 in]
                        n232 = Concatenate Strings(w571, w570, ";" ("string")) -> (w565:string)
                      }
                      frame "Returns the string AS auto-restart mode status" {
                        n233 = Index Array(array=w588, index=w589) -> (element=w587:string)
                      }
                    }
                  }
                }
              }
              frame #2 {
                n234 = case shown="True" w591 {
                  tunnel: w594 -> [w596 w601]
                  tunnel: w593 -> [w595 w600]
                  tunnel: w590 -> [_ w599]
                  tunnel: [w596 w598] -> _
                  tunnel: [w595 w597] -> w592
                  frame False {
                  }
                  frame True {
                    n235 = VISA Write(VISA resource name=w601, write buffer=w599, error in (no error)=w600) -> (VISA resource name out=w598:refnum<visa-resource-name>, error out=w597:errorcluster)  [unwired: 1 out]
                  }
                }
                n236 = property on="Code 2" class="Str"("Value"=w590) -> ()  [unwired: 2 in, 2 out]
              }
            }
          }
        }
        n237 = Unbundle By Name(w20) -> ("status"=w25:bool)
        n238 = Or(x=w24, y=w25) -> (x .or. y?=w23:bool)
      }
    }
    frame #2 {
      n239 = VISA Close(VISA resource name=w604, error in (no error)=w603) -> (error out=w602:errorcluster)
      n240 = call <vilib>:"Simple Error Handler.vi"("error in (no error)"=w602) -> ()  [unwired: 4 in, 5 out]
    }
  }
